vi "Import Digital Pattern File.vi"(8 "error in (no error)":errorcluster) -> (0 "error out":errorcluster, 2 "Canceled?":bool, 3 "EPT Pattern":T1)   [LabVIEW 2020, in "Engine Simulation Toolkit System Explorer.lvlib"]
uses:
  Engine Simulation Toolkit System Explorer.lvlib
  File Formats.lvlibp/Parent/EST Pattern.ctl
  File Formats.lvlibp/Parent/FileFormat.lvclass
panel:
  in  "Cancel":bool
  in  "OK":bool
  in  "Path":path
  in  "Format":string(combo)
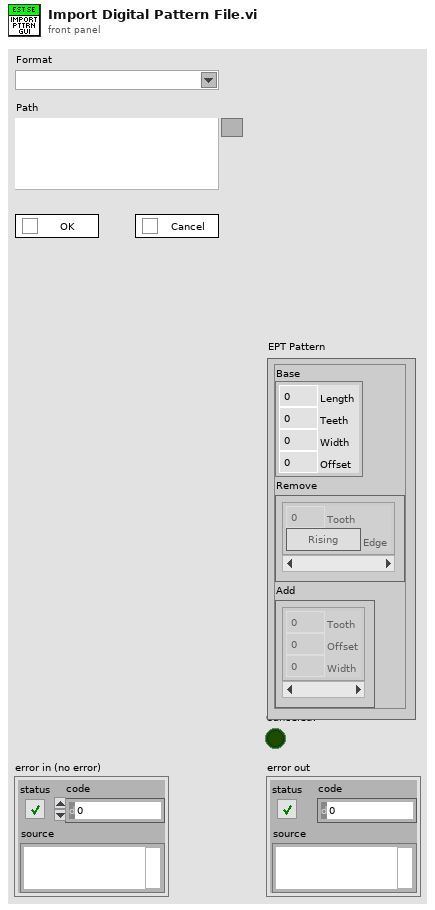
[diagram p1: front panel]
types:
  T1 = typedef "File Formats.lvlibp/FileFormat.lvclass/EST Pattern.ctl" = cluster{"Base":cluster{"Length":dbl, "Teeth":u16, "Width":dbl, "Offset":dbl}, "Remove":cluster{"Tooth":u16, "Edge":bool}[], "Add":cluster{"Tooth":u16, "Offset":dbl, "Width":dbl}[]}
  T2 = enum8{"Enabled", "Disabled", "Disabled and Grayed Out"}
  T3 = typedef "File Formats.lvlibp/FileFormat.lvclass/Extension Info.ctl" = cluster{"Value":string, "Tag":string}
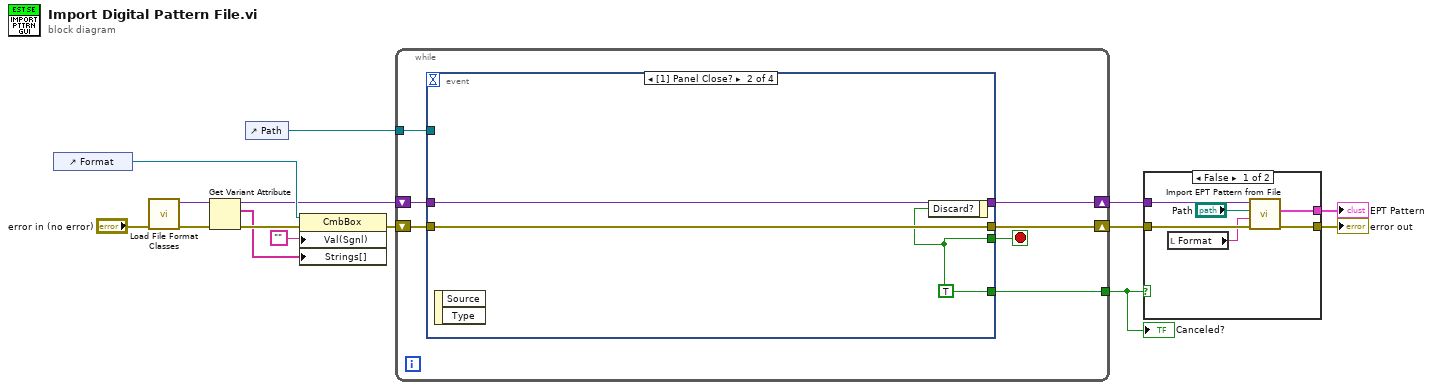
[diagram p0: block diagram]
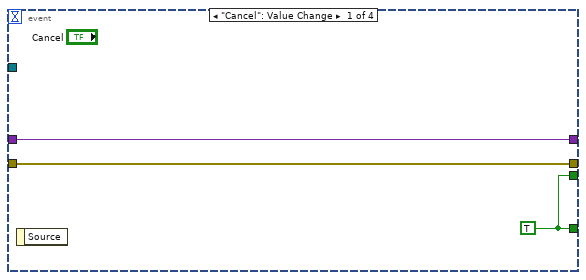
[diagram p3: hidden frame]
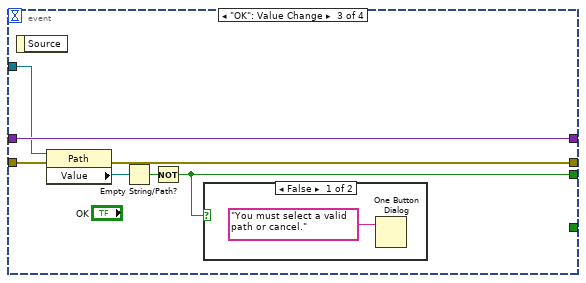
[diagram p4: hidden frame]
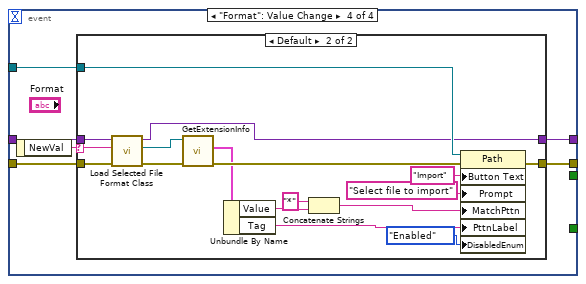
[diagram p6: hidden frame]
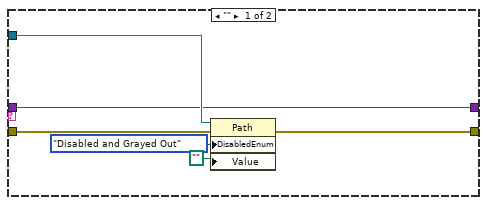
[diagram p7: hidden frame]
diagram:
  n1 = control-ref of="Format"() -> (w14:refnum<vi>)
  n2 = call "Load File Format Classes.vi"("error in (no error)"="error in (no error)") -> ("error out"=w9:errorcluster, "Class Lookup"=w10:variant)  [unwired: 9 in]
  n3 = Get Variant Attribute(Variant=w10, error in=w9) -> (duplicate Variant=w4:variant, names=w7:string[], error out=w8:errorcluster)  [unwired: 2 in, 1 out]
  n4 = control-ref of="Path"() -> (w15:refnum<vi>)
  n5 = property class="CmbBox"(reference=w14, error in=w8, "Val(Sgnl)"="", "Strings[]"=w7) -> (error out=w13:errorcluster)  [unwired: 1 out]
  n6 = while {
    tunnel: w15 -> [w22]
    shift-right: [w18] -> w3
    shift-left: w4 -> [w19]
    shift-right: [w20] -> w5
    shift-left: w13 -> [w21]
    tunnel: [w16] -> w1
    stop <- w17 stop-if-true
    n7 = event shown="[1] Panel Close?" {
      selector: _ -> [_ _ _ _]
      dyn-events: _ -> [_ _ _ _]
      timeout: _ -> [_ _ _ _]
      tunnel: w22 -> [_ _ w34 w42]
      tunnel: [w25 w28 w32 w41] -> w20
      tunnel: w21 -> [w25 w28 w33 w39]
      tunnel: w19 -> [w24 w27 w35 w38]
      tunnel: [w24 w27 w35 w37] -> w18
      tunnel: [w23 w26 w29 _] -> w17
      tunnel: [w23 w26 _ _] -> w16
      event "Cancel": Value Change {
        w23 = TRUE
        n8 = event-data() -> ()  [unwired: 1 in, 1 out]
      }
      event Panel Close? {
        w26 = TRUE
        n9 = event-data() -> ()  [unwired: 1 in, 2 out]
        n10 = event-data("Discard?"=w26) -> ()  [unwired: 1 in, 1 out]
      }
      event "OK": Value Change {
        n11 = event-data() -> ()  [unwired: 1 in, 1 out]
        n12 = property class="Path"(reference=w34, error in=w33) -> (error out=w32:errorcluster, "Value"=w31:path)  [unwired: 1 out]
        n13 = Empty String/Path?(string/path=w31) -> (empty?=w30:bool)
        n14 = Not(x=w30) -> (.not. x?=w29:bool)
        n15 = case shown="False" w29 {
          frame False {
            n16 = One Button Dialog(message="You must select a valid path or cancel.") -> ()  [unwired: 1 in, 1 out]
          }
          frame True {
          }
        }
      }
      event "Format": Value Change {
        n17 = event-data() -> ("NewVal"=w40:string)  [unwired: 1 in]
        n18 = case shown="Default" w40 {
          selector: w40 -> [_ w52]
          tunnel: w42 -> [w46 w64]
          tunnel: [w47 w56] -> w41
          tunnel: w39 -> [w44 w54]
          tunnel: w38 -> [w43 w51]
          tunnel: [w43 w49] -> w37
          frame "" {
            n19 = property class="Path"(reference=w46, error in=w44, "DisabledEnum"=T2."Disabled and Grayed Out" ("Disabled"), "Value"=path "") -> (error out=w47:errorcluster)  [unwired: 1 out]
          }
          frame Default {
            n20 = call "Load Selected File Format Class.vi"("error in (no error)"=w54, "Protocol in"=w52, "Class Lookup"=w51) -> ("error out"=w53:errorcluster, "FileFormat.lvclass"=w50:refnum<class "FileFormat.lvclass">, "Class Lookup"=w49:variant)  [unwired: 6 in]
            n21 = call-dynamic "GetExtensionInfo.vi"("error in (no error)"=w53, "FileFormat in"=w50) -> ("error out"=w63:errorcluster, "Extension Info"=w62:T3)  [unwired: 7 in, 1 out]
            n22 = Unbundle By Name(w62) -> ("Value"=w61:string, "Tag"=w58:string)
            n23 = Concatenate Strings("*" ("string"), w61) -> (w59:string)
            n24 = property class="Path"(reference=w64, error in=w63, "Button Text"="Import" ("Browse Options:Button Text"), "Prompt"="Select file to import" ("Browse Options:Button Text"), "MatchPttn"=w59, "PttnLabel"=w58, "DisabledEnum"=T2."Enabled" ("Disabled")) -> (error out=w56:errorcluster)  [unwired: 1 out]
          }
        }
      }
    }
  }
  "Canceled?" <- w1
  n25 = case shown="False" w1 {
    tunnel: [w71 w72] -> w6
    tunnel: w5 -> [w70 w72]
    tunnel: w3 -> [w69 _]
    tunnel: [w68 _] -> w2
    frame False {
      n26 = local read "Format"() -> (w66:string)
      n27 = call "Import EPT Pattern from File.vi"("error in (no error)"=w70, "Protocol in"=w66, "Path"="Path", "Class Lookup"=w69) -> ("error out"=w71:errorcluster, "EPT Pattern"=w68:T1)  [unwired: 5 in, 1 out]
    }
    frame True {
    }
  }
  "error out" <- w6
  "EPT Pattern" <- w2
